vi "GraphConfCount.vi"(8 "error in (no error)":errorcluster caption="entrée d'erreur", 9 "Configuration":i32) -> (0 "error out":errorcluster caption="sortie d'erreur", 2 "GraphCount":i32)   [LabVIEW 2010]
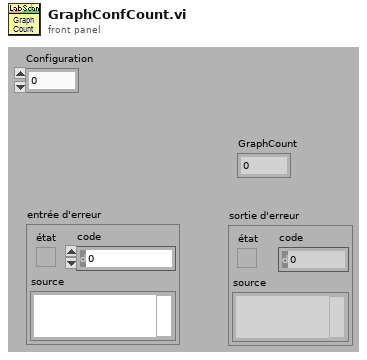
[diagram p1: front panel]
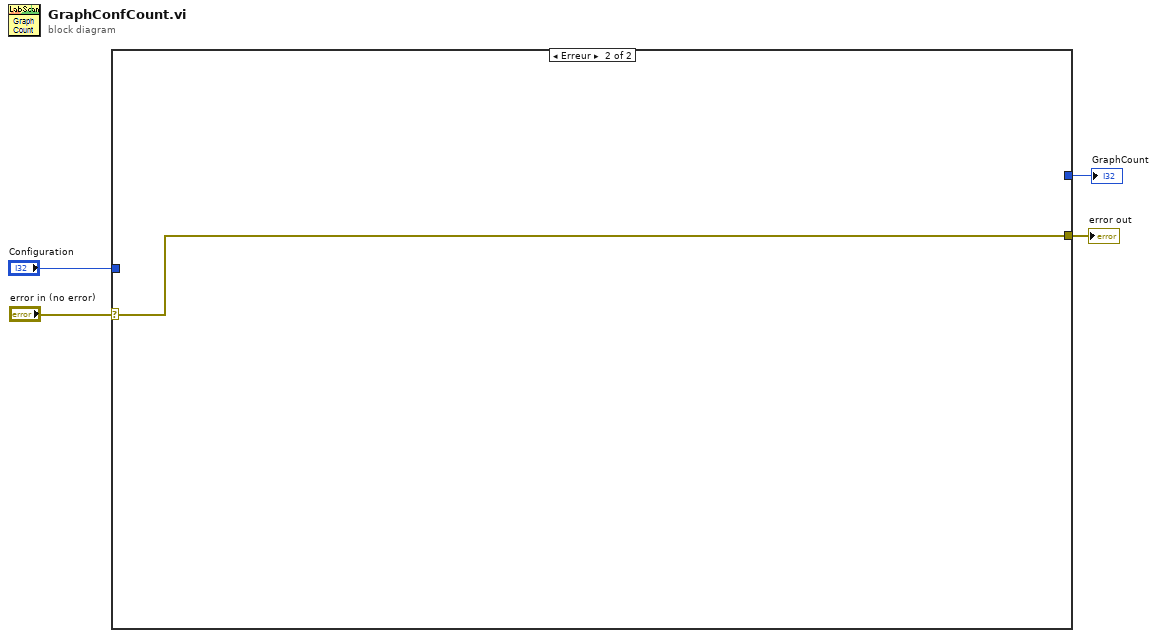
[diagram p0: block diagram]
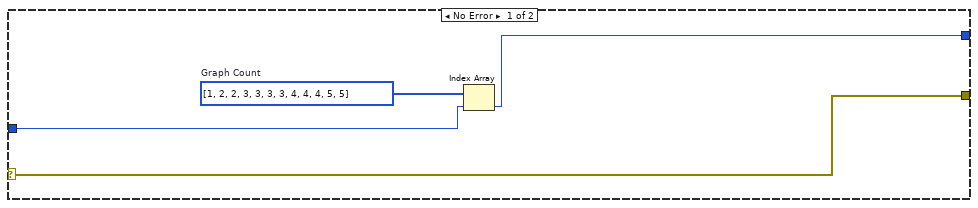
[diagram p2: hidden frame]
diagram:
  n1 = case shown="Erreur" "error in (no error)" {
    selector: "error in (no error)" -> [w6 w9]
    tunnel: "Configuration" -> [w7 _]
    tunnel: [w6 w9] -> w3
    tunnel: [w5 _] -> w1
    frame No Error {
      w8 = i32[] [1, 2, 2, 3, 3, 3, 3, 4, 4, 4, 5, 5]  # Graph Count
      n2 = Index Array(array=w8, index=w7) -> (element=w5:i32)
    }
    frame Error {
    }
  }
  "error out" <- w3
  "GraphCount" <- w1
